vi "Software Update HCC Update Config File.vi"(4 "Station Name":string, 6 "Updated Input":string[](array[string]), 8 "Error In":errorcluster, 9 "Station index":u32, 10 "Newfi Exe Locations":path, 11 "Newfi Exe Folder Path":path) -> (0 "Error Out":errorcluster, 2 "Updated Configuration File":string[][](array[string]), 3 "Configuration File":string[][](array[string]))   [LabVIEW 2016]
uses:
  <vilib>/Utility/file.llb/Read Delimited Spreadsheet (string).vi
  <vilib>/Utility/file.llb/Write Delimited Spreadsheet (string).vi
panel:
  out "element":string
  out "appended path":path
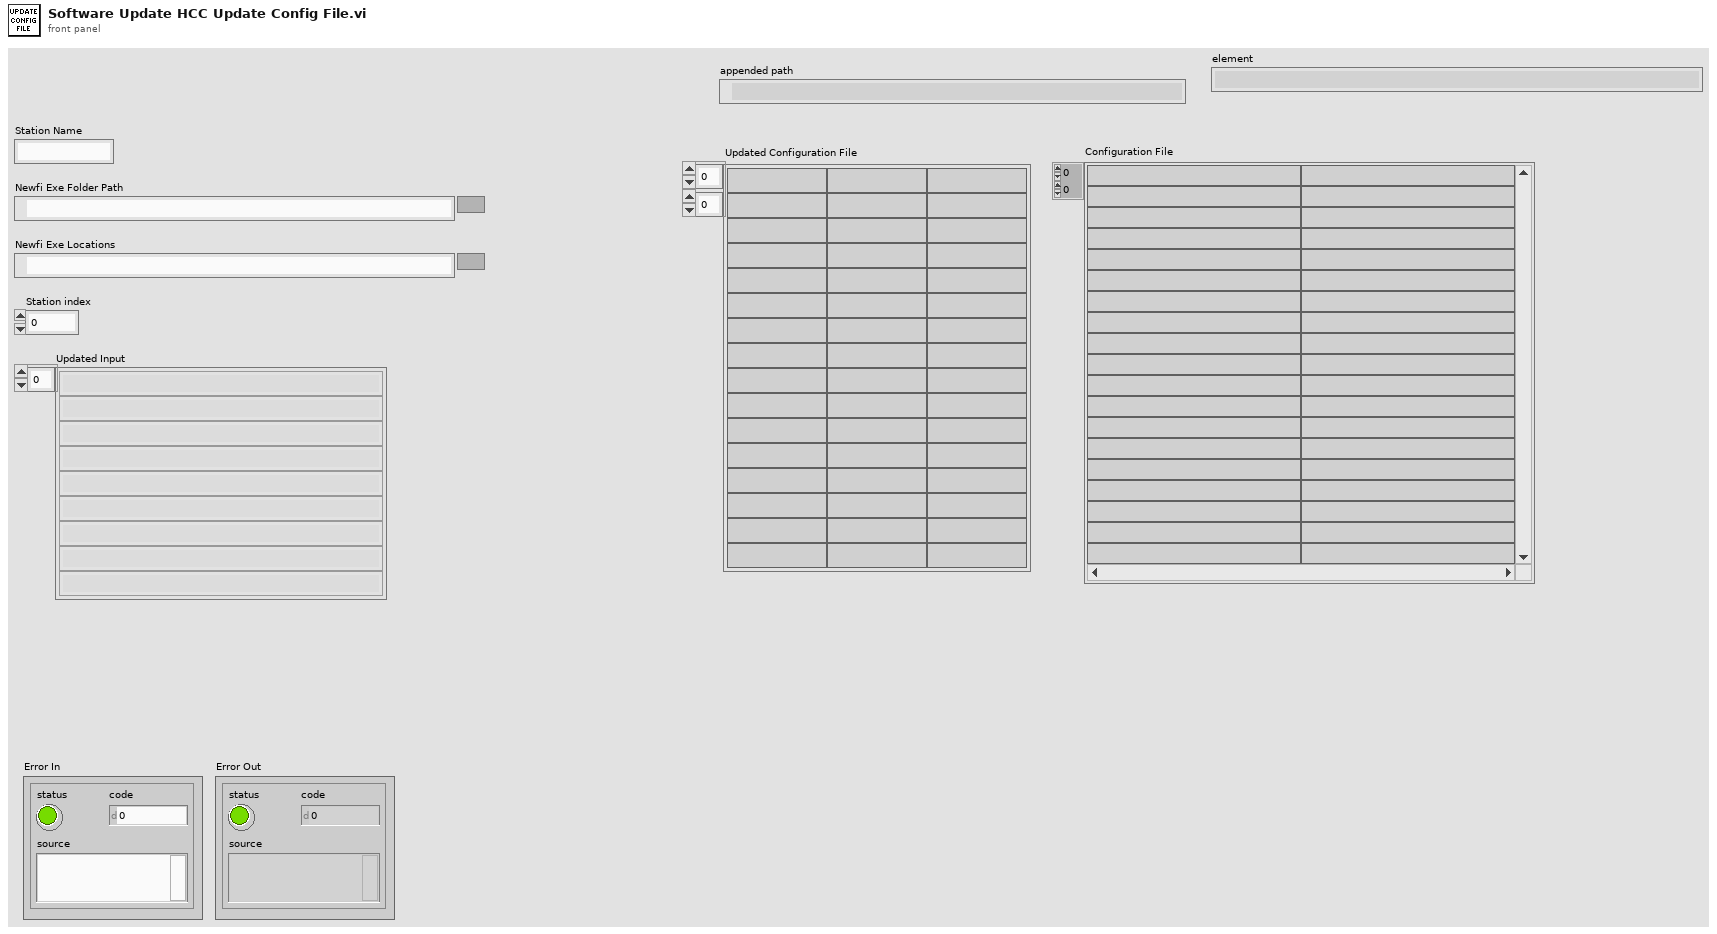
[diagram p1: front panel]
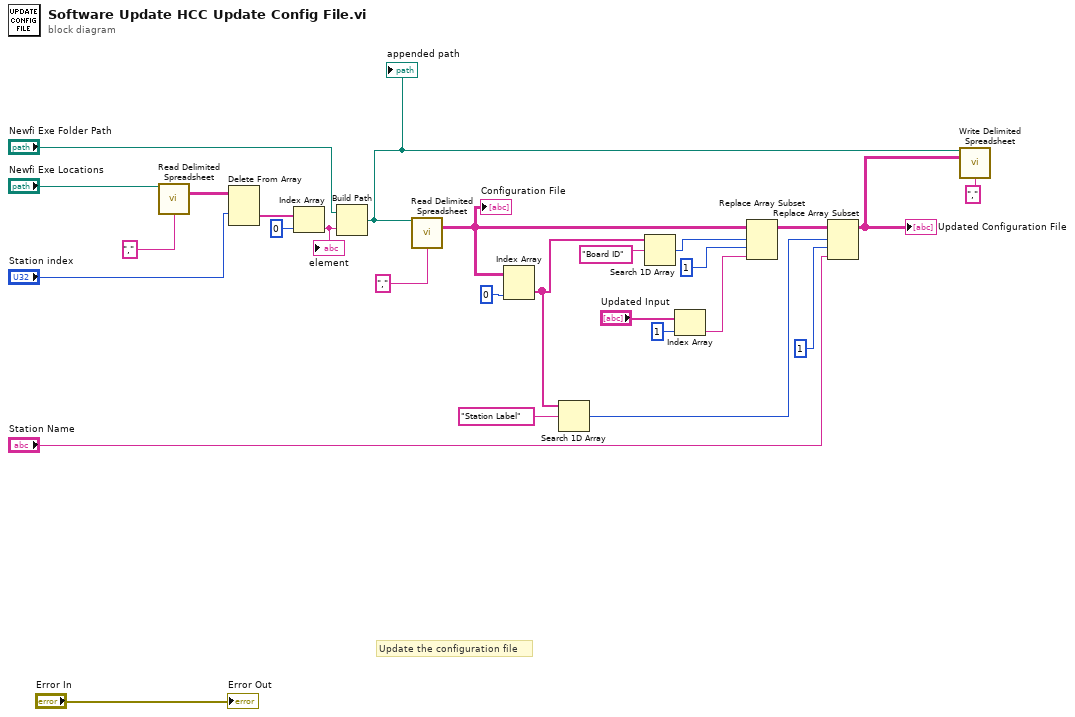
[diagram p0: block diagram]
diagram:
  # "Update the configuration file"
  n1 = call-poly <vilib>:"Read Delimited Spreadsheet.vi"("file path (dialog if empty)"="Newfi Exe Locations", "delimiter (\\t)"="," ("delimiter (\\t)")) -> ("all rows"=w18:string[][])  [unwired: 8 in, 5 out]
  n2 = Delete From Array(array=w18, index (row)="Station index") -> (deleted portion=w2:string[])  [unwired: 2 in, 1 out]
  n3 = Index Array(array=w2, index=0) -> (element=w26:string)
  "element" <- w26
  n4 = Build Path(base path="Newfi Exe Folder Path", name or relative path=w26) -> (appended path=w27:path)
  "appended path" <- w27
  n5 = call-poly <vilib>:"Read Delimited Spreadsheet.vi"("file path (dialog if empty)"=w27, "delimiter (\\t)"="," ("delimiter (\\t)")) -> ("all rows"=w21:string[][])  [unwired: 8 in, 5 out]
  "Configuration File" <- w21
  n6 = Index Array(array=w21, index (col)=0 ("disabled index (col)")) -> (element=w6:string[])  [unwired: 1 in]
  n7 = Search 1D Array(1D array=w6, element="Station Label") -> (index of element=w11:i32)  [unwired: 1 in]
  n8 = Search 1D Array(1D array=w6, element="Board ID") -> (index of element=w13:i32)  [unwired: 1 in]
  n9 = Index Array(array="Updated Input", index=1) -> (element=w15:string)
  n10 = Replace Array Subset(array=w21, new element=w15, index (row)=w13, index (col)=1 ("disabled index (col)")) -> (w14:string[][])
  n11 = Replace Array Subset(array=w14, new element="Station Name", index (row)=w11, index (col)=1 ("disabled index (col)")) -> (w22:string[][])
  "Updated Configuration File" <- w22
  n12 = call-poly <vilib>:"Write Delimited Spreadsheet.vi"("file path (dialog if empty)"=w27, "2D data"=w22, "delimiter (\\t)"="," ("delimiter (\\t)")) -> ()  [unwired: 11 in, 2 out]
  "Error Out" <- "Error In"
